vi "Vector_Plotting.vi"(1 "JobVectorDirectory":path, 2 "Data":string[][](array[string]), 3 "Template Filename":path, 4 "Channel Names":string[](array[string])) -> ()   [LabVIEW 2013]
uses:
  Controls/Group_Binning.ctl
  Data_File_Type.ctl
panel:
  in  "Plot scalar Values":bool
  in  "V":u16(ring) items=["Comment", "Azimuth", "BoomHt", "X (mm)", "Y (mm)", "Z (mm)", "Uref (m/s)", "Utest (m/s)", "U/Uref", "V/Uref", "W/Uref", "Vmag5HP/Uref", "TI(U) (%)", "TI(V) (%)", "TI(W) (%)", "TI(Vmag) (%)", "GoodFraction", "U", "U_Var", "V", "V_Var", "W", "W_Var", "Vmag", "Vmag_Var", "5HP-1 Mean mmH2O", "5HP-2 Mean mmH2O", "5HP-3 Mean mmH2O", "5HP-4 Mean mmH2O", "5HP-5 Mean mmH2O", "5HP-1 Timescale", "5HP-2 Timescale", "5HP-3 Timescale", "5HP-4 Timescale", "5HP-5 Timescale", "Z(Uref) (mm)", "Spires", "Trip", "RoughnessHeight", "RoughnessLength", "AdditionalElements", "TTSetup", "Date of Measurement", "MultiRun Start Time", "Meas Time", "Time Stamp", "Run Messages", "Row Type", "Measurement Type", "Av Analogue Sampling Rate", "No of Analogue Samples", "No Of Measurement Blocks", "Flow Measurement Time", "Reference Temperature Used for Corrections", "Mano (5HP-1) Calibration Filename", "Mano (5HP-2) Calibration Filename", "Mano (5HP-3) Calibration Filename", "Mano (5HP-4) Calibration Filename", "Mano (5HP-5) Calibration Filename", "Original Results Filename", "Current Data Filename", "Raw Data Filename", "Multi Run Row Number"]
  in  "U":u16(ring) items=["Comment", "Azimuth", "BoomHt", "X (mm)", "Y (mm)", "Z (mm)", "Uref (m/s)", "Utest (m/s)", "U/Uref", "V/Uref", "W/Uref", "Vmag5HP/Uref", "TI(U) (%)", "TI(V) (%)", "TI(W) (%)", "TI(Vmag) (%)", "GoodFraction", "U", "U_Var", "V", "V_Var", "W", "W_Var", "Vmag", "Vmag_Var", "5HP-1 Mean mmH2O", "5HP-2 Mean mmH2O", "5HP-3 Mean mmH2O", "5HP-4 Mean mmH2O", "5HP-5 Mean mmH2O", "5HP-1 Timescale", "5HP-2 Timescale", "5HP-3 Timescale", "5HP-4 Timescale", "5HP-5 Timescale", "Z(Uref) (mm)", "Spires", "Trip", "RoughnessHeight", "RoughnessLength", "AdditionalElements", "TTSetup", "Date of Measurement", "MultiRun Start Time", "Meas Time", "Time Stamp", "Run Messages", "Row Type", "Measurement Type", "Av Analogue Sampling Rate", "No of Analogue Samples", "No Of Measurement Blocks", "Flow Measurement Time", "Reference Temperature Used for Corrections", "Mano (5HP-1) Calibration Filename", "Mano (5HP-2) Calibration Filename", "Mano (5HP-3) Calibration Filename", "Mano (5HP-4) Calibration Filename", "Mano (5HP-5) Calibration Filename", "Original Results Filename", "Current Data Filename", "Raw Data Filename", "Multi Run Row Number"]
  in  "Y Axis":u16(ring) items=["Comment", "Azimuth", "BoomHt", "X (mm)", "Y (mm)", "Z (mm)", "Uref (m/s)", "Utest (m/s)", "U/Uref", "V/Uref", "W/Uref", "Vmag5HP/Uref", "TI(U) (%)", "TI(V) (%)", "TI(W) (%)", "TI(Vmag) (%)", "GoodFraction", "U", "U_Var", "V", "V_Var", "W", "W_Var", "Vmag", "Vmag_Var", "5HP-1 Mean mmH2O", "5HP-2 Mean mmH2O", "5HP-3 Mean mmH2O", "5HP-4 Mean mmH2O", "5HP-5 Mean mmH2O", "5HP-1 Timescale", "5HP-2 Timescale", "5HP-3 Timescale", "5HP-4 Timescale", "5HP-5 Timescale", "Z(Uref) (mm)", "Spires", "Trip", "RoughnessHeight", "RoughnessLength", "AdditionalElements", "TTSetup", "Date of Measurement", "MultiRun Start Time", "Meas Time", "Time Stamp", "Run Messages", "Row Type", "Measurement Type", "Av Analogue Sampling Rate", "No of Analogue Samples", "No Of Measurement Blocks", "Flow Measurement Time", "Reference Temperature Used for Corrections", "Mano (5HP-1) Calibration Filename", "Mano (5HP-2) Calibration Filename", "Mano (5HP-3) Calibration Filename", "Mano (5HP-4) Calibration Filename", "Mano (5HP-5) Calibration Filename", "Original Results Filename", "Current Data Filename", "Raw Data Filename", "Multi Run Row Number"]
  in  "X Axis":u16(ring) items=["Comment", "Azimuth", "BoomHt", "X (mm)", "Y (mm)", "Z (mm)", "Uref (m/s)", "Utest (m/s)", "U/Uref", "V/Uref", "W/Uref", "Vmag5HP/Uref", "TI(U) (%)", "TI(V) (%)", "TI(W) (%)", "TI(Vmag) (%)", "GoodFraction", "U", "U_Var", "V", "V_Var", "W", "W_Var", "Vmag", "Vmag_Var", "5HP-1 Mean mmH2O", "5HP-2 Mean mmH2O", "5HP-3 Mean mmH2O", "5HP-4 Mean mmH2O", "5HP-5 Mean mmH2O", "5HP-1 Timescale", "5HP-2 Timescale", "5HP-3 Timescale", "5HP-4 Timescale", "5HP-5 Timescale", "Z(Uref) (mm)", "Spires", "Trip", "RoughnessHeight", "RoughnessLength", "AdditionalElements", "TTSetup", "Date of Measurement", "MultiRun Start Time", "Meas Time", "Time Stamp", "Run Messages", "Row Type", "Measurement Type", "Av Analogue Sampling Rate", "No of Analogue Samples", "No Of Measurement Blocks", "Flow Measurement Time", "Reference Temperature Used for Corrections", "Mano (5HP-1) Calibration Filename", "Mano (5HP-2) Calibration Filename", "Mano (5HP-3) Calibration Filename", "Mano (5HP-4) Calibration Filename", "Mano (5HP-5) Calibration Filename", "Original Results Filename", "Current Data Filename", "Raw Data Filename", "Multi Run Row Number"]
  in  "OK Button":bool
  in  "Row Selector":i32(listbox)=1
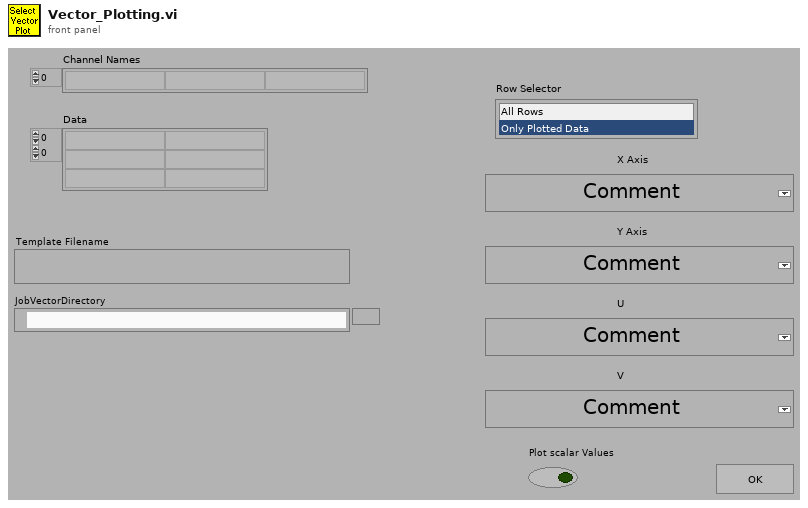
[diagram p1: front panel]
types:
  T1 = typedef "Data_File_Type.ctl" = enum16{"Read All File Types", "Results Files Only", "Raw Data Files Only", "Calibration Files Only", "Gas Desk Files Only", "Old Results Files Only", "Tabulated Data Files Only"}
  T2 = enum16{"Show only data summary", "Show data summary", "No data summary"}
  T3 = typedef "Group_Binning.ctl" = cluster{"Index":i32, "Tolerance":dbl, "Precision":string}
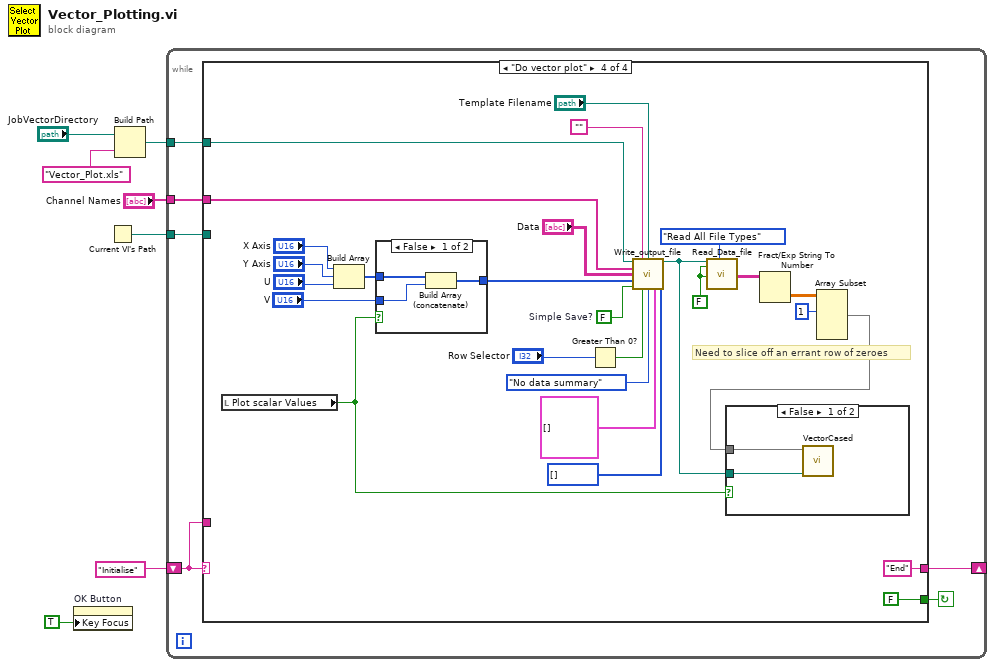
[diagram p0: block diagram]
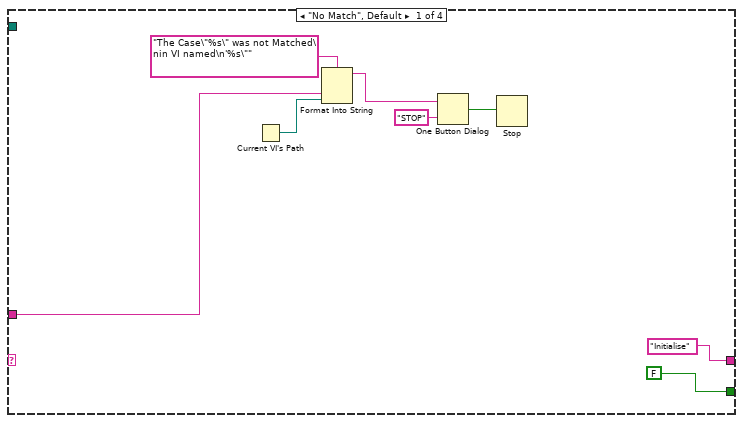
[diagram p2: hidden frame]
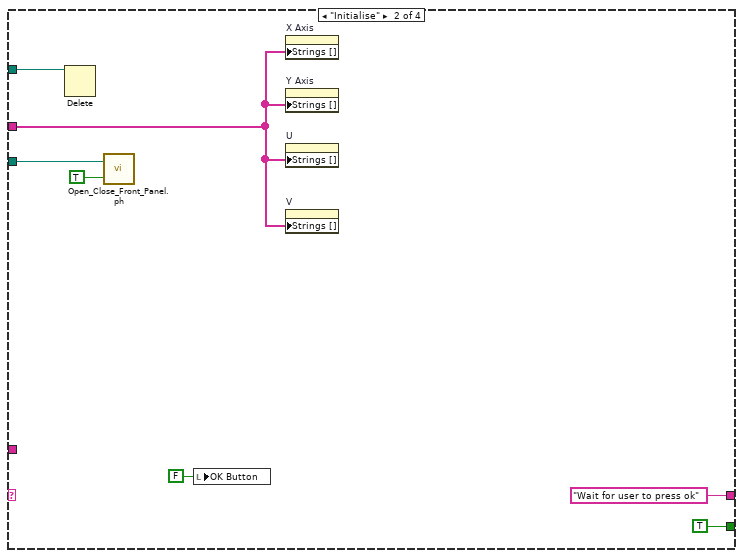
[diagram p3: hidden frame]
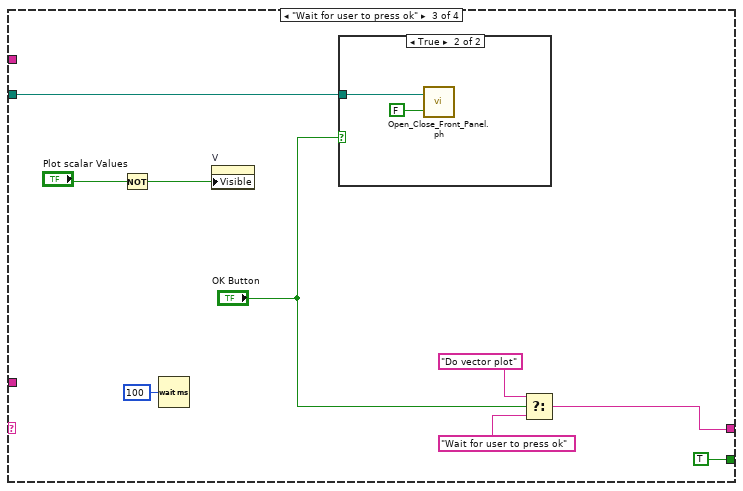
[diagram p4: hidden frame]
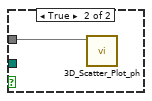
[diagram p6: hidden frame]
diagram:
  n1 = property on="OK Button" class="Bool (strict)"("Key Focus"=TRUE) -> ()  [unwired: 2 in, 2 out]
  n2 = Current VI's Path() -> (path=w6:path)
  n3 = Build Path(base path="JobVectorDirectory", name or relative path="Vector_Plot.xls") -> (appended path=w1:path)
  n4 = while {
    shift-left: "Initialise" -> [w11]
    shift-right: [w12] -> _
    tunnel: w6 -> [w10]
    tunnel: "Channel Names" -> [w9]
    tunnel: w1 -> [w8]
    stop <- w13 continue-if-true
    n5 = case shown="\"Do vector plot\"" w11 {
      tunnel: [FALSE TRUE TRUE FALSE] -> w13
      tunnel: ["Initialise" "Wait for user to press ok" w36 "End" ("t")] -> w12
      tunnel: w11 -> [w16 _ _ _]
      tunnel: w10 -> [_ w26 w31 _]
      tunnel: w9 -> [_ w24 _ w50]
      tunnel: w8 -> [_ w22 _ w49]
      frame "No Match", Default {
        n6 = Current VI's Path() -> (path=w15:path)
        n7 = Format Into String(format string="The Case\"%s\" was not Matched\nin VI named\n'%s\"" ("Format String"), w16, w15) -> (resulting string=w19:string)  [unwired: 2 in, 1 out]
        n8 = One Button Dialog(message=w19, button name ("OK")="STOP") -> (true=w17:bool)
        n9 = Stop(stop? (T)=w17) -> ()
      }
      frame "Initialise" {
        n10 = Delete(path (use dialog)=w22) -> ()  [unwired: 1 in, 6 out]
        n11 = call "Open_Close_Front_Panel.ph.vi"("Front Panel Window:Open"=TRUE, "VI path"=w26) -> ()  [unwired: 2 out]
        n12 = local write "OK Button"(FALSE ("OK Button")) -> ()
        n13 = property on="X Axis" class="Ring (strict)"("Strings []"=w24) -> ()  [unwired: 2 in, 2 out]
        n14 = property on="Y Axis" class="Ring (strict)"("Strings []"=w24) -> ()  [unwired: 2 in, 2 out]
        n15 = property on="U" class="Ring (strict)"("Strings []"=w24) -> ()  [unwired: 2 in, 2 out]
        n16 = property on="V" class="Ring (strict)"("Strings []"=w24) -> ()  [unwired: 2 in, 2 out]
      }
      frame "Wait for user to press ok" {
        n17 = Not(x="Plot scalar Values") -> (.not. x?=w29:bool)
        n18 = Wait (ms)(milliseconds to wait=u32 100) -> ()  [unwired: 1 out]
        n19 = property on="V" class="Ring (strict)"("Visible"=w29) -> ()  [unwired: 2 in, 2 out]
        n20 = case shown="True" "OK Button" {
          tunnel: w31 -> [_ w38]
          frame False {
          }
          frame True {
            n21 = call "Open_Close_Front_Panel.ph.vi"("Front Panel Window:Open"=FALSE, "VI path"=w38) -> ()  [unwired: 2 out]
          }
        }
        n22 = Select(t="Do vector plot", s="OK Button", f="Wait for user to press ok") -> (s? t:f=w36:string)
      }
      frame "Do vector plot" {
        w53 = FALSE ("Read Channel Names only")
        w59 = FALSE  # Simple Save?
        # "Need to slice off an errant row of zeroes"
        n23 = local read "Plot scalar Values"() -> (w41:bool)
        n24 = Build Array("X Axis", "Y Axis", "U") -> (w44:u16[])
        n25 = case shown="False" w41 {
          tunnel: w44 -> [w72 w73]
          tunnel: "V" -> [w71 _]
          tunnel: [w70 w73] -> w42
          frame False {
            n26 = Build Array (concatenate)(w72, w71) -> (w70:u16[])
          }
          frame True {
          }
        }
        n27 = Greater Than 0?(x="Row Selector") -> (x > 0?=w60:bool)
        n28 = call "Write_output_file.vi"("Output filename"=w49, "Header"="", "Template Filename"="Template Filename", "Channel Names"=w50, "Data"="Data", "Desired Columns"=w42, "Simple Save?"=w59, "Save Plotted rows only?"=w60, "Summarise mode"=T2."No data summary", "Grouping info"=T3[] [], "Channels to Tabulate in header"=i32[] []) -> ("Output filename Out"=w40:path)  [unwired: 1 in, 3 out]
        n29 = call "Read_Data_file.vi"("Results file"=w40, "Read Channel Names only"=w53, "Add Extra Channels?"=w53, "Desired File Types"=Data_File_Type."Read All File Types") -> ("Channel Values Out"=w51:string[][])  [unwired: 1 in, 14 out]
        n30 = Fract/Exp String To Number(string=w51) -> (number=w47:dbl[][])  [unwired: 4 out]
        n31 = Array Subset(array=w47, index (row)=1 ("index")) -> (w46:dbl[][])  [unwired: 3 in]
        n32 = case shown="False" w41 {
          tunnel: w46 -> [w68 w69]
          tunnel: w40 -> [w67 _]
          frame False {
            n33 = call "VectorCased.vi"("DatafileLocation"=w67, "XYUVArray"=w68) -> ()  [unwired: 10 out]
          }
          frame True {
            n34 = call "3D_Scatter_Plot_ph.vi"("XYUVArray"=w69) -> ()  [unwired: 11 in]
          }
        }
      }
    }
  }
